vi "Read Stage Position.vi"(8 "error in (no error)":errorcluster, 11 "MAS in":refnum<class "MAS.lvclass">) -> (0 "error out":errorcluster, 2 "Position":dbl[](array[numeric]), 3 "MAS out":refnum<class "MAS.lvclass">)   [LabVIEW 2022 SP3, in "MAS.lvclass"]
uses:
  MAS.lvclass
  MAS.lvclass/MAS.ctl
  iMotion Controller/iMotion Controller.lvclass
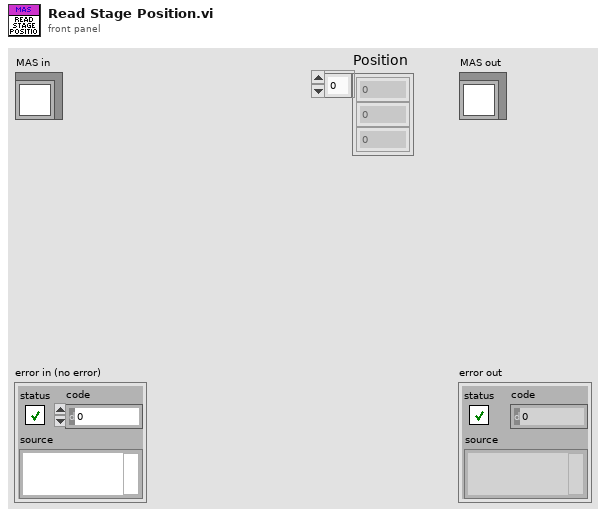
[diagram p1: front panel]
types:
  T1 = map{string, refnum<class "iMotion Controller.lvclass">}
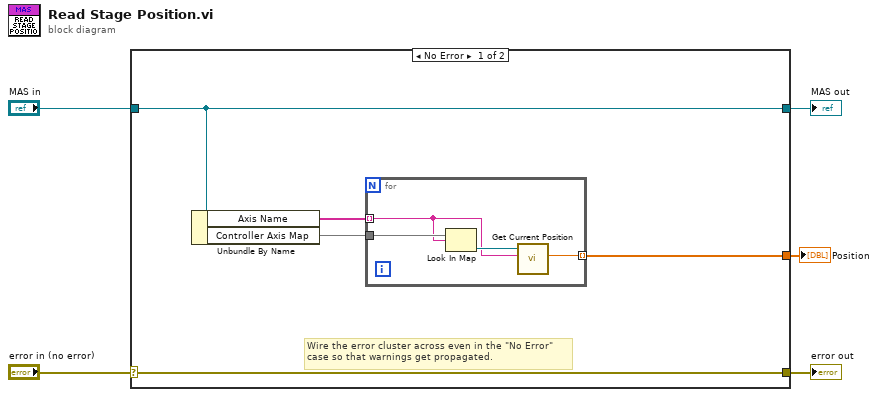
[diagram p0: block diagram]
diagram:
  n1 = case shown="No Error" "error in (no error)" {
    selector: "error in (no error)" -> [w10 w16]
    tunnel: [w10 w16] -> w4
    tunnel: [w9 w15] -> w2
    tunnel: "MAS in" -> [w9 w15]
    tunnel: [w6 _] -> w1
    frame No Error {
      # "Wire the error cluster across even in the \"No Error\"\ncase so that warnings get propagated."
      n2 = Unbundle By Name(w9) -> ("Axis Name"=w8:string[], "Controller Axis Map"=w7:T1)
      n3 = for {
        tunnel: w8 -> [w12] mode=indexing
        tunnel: w7 -> [w14]
        tunnel: [w11] -> w6 mode=indexing
        n4 = Look In Map(map=w14, key=w12) -> (value=w13:refnum<class "iMotion Controller.lvclass">)  [unwired: 1 in, 1 out]
        n5 = call-dynamic "Get Current Position.vi"("Axis Name"=w12, "iMotion Controller in"=w13) -> ("Current Position"=w11:dbl)  [unwired: 7 in, 2 out]
      }
    }
    frame Error {
    }
  }
  "error out" <- w4
  "MAS out" <- w2
  "Position" <- w1
